vi "convert_voltage_to_motech.vi"(8 "error_in":errorcluster, 10 "determined_channels":T3, 11 "voltage":dbl) -> (0 "error_out":errorcluster, 3 "motech_set_value":T1)   [LabVIEW 2017]
uses:
  types/channels_enum.ctl
  types/motech_set_value_cluster.ctl
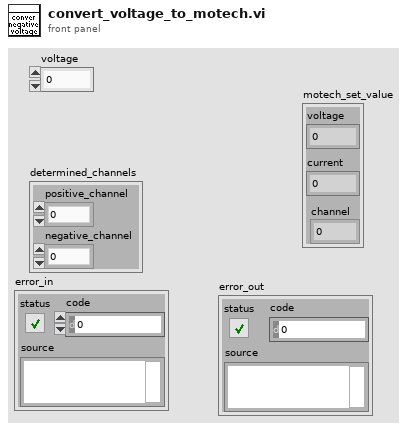
[diagram p1: front panel]
types:
  T1 = typedef "motech_set_value_cluster.ctl" = cluster{"voltage":dbl, "current":dbl, "channel":T2}
  T2 = typedef "channels_enum.ctl" = enum16{"0", "1", "2"}
  T3 = cluster{"positive_channel":T2, "negative_channel":T2}
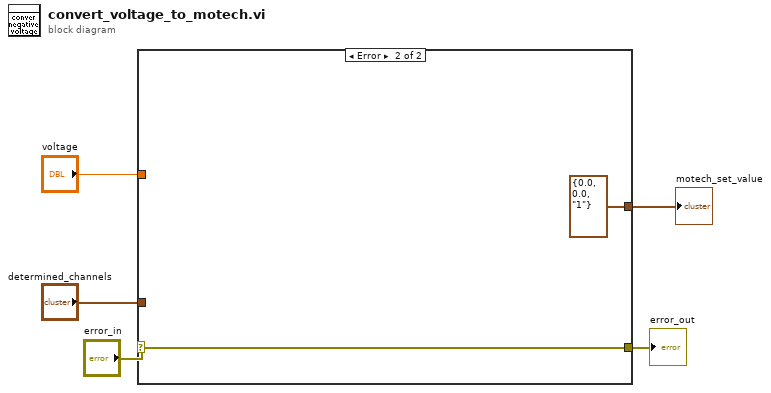
[diagram p0: block diagram]
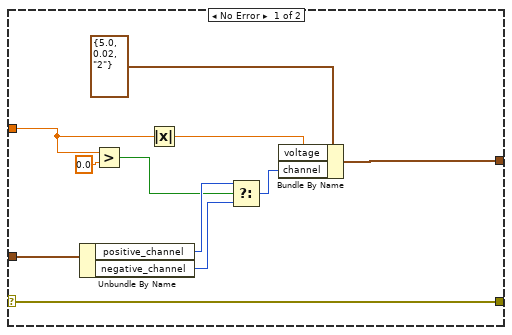
[diagram p2: hidden frame]
diagram:
  n1 = case shown="Error" "error_in" {
    selector: "error_in" -> [w6 w18]
    tunnel: "determined_channels" -> [w13 _]
    tunnel: "voltage" -> [w11 _]
    tunnel: [w9 T1 {"voltage"=0.0, "current"=0.0, "channel"=enum."1"} ("motech_set_value")] -> w3
    tunnel: [w6 w18] -> w2
    frame No Error {
      n2 = Unbundle By Name(w13) -> ("positive_channel"=w14:T2, "negative_channel"=w15:T2)
      n3 = Greater?(x=w11, y=0.0) -> (0:w12:bool)
      n4 = Absolute Value(x=w11) -> (abs(x)=w10:dbl)
      n5 = Select(t=w14, s=w12, f=w15) -> (s? t:f=w16:T2)
      n6 = Bundle By Name(cluster=T1 {"voltage"=5.0, "current"=0.02, "channel"=enum."2"} ("motech_set_value"), "voltage"=w10, "channel"=w16) -> (w9:T1)
    }
    frame Error {
    }
  }
  "motech_set_value" <- w3
  "error_out" <- w2
